vi "Send home.vi"(8 "error in (no error)":errorcluster, 11 "FCR Mod ID":i32) -> (0 "error out":errorcluster, 3 "Home?":bool)   [LabVIEW 2020]
uses:
  Newport_FCR100/Libraries/FCR100/Support/Device state -- enum.ctl
  Newport_FCR100/Libraries/FCR100/FCR100.lvlib
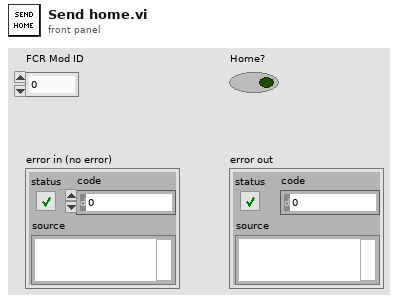
[diagram p1: front panel]
types:
  T1 = typedef "FCR100.lvlib/Device state -- enum.ctl" = enum16{"Not referenced", "Configuration", "Disable", "Ready", "Homing", "Motion"}
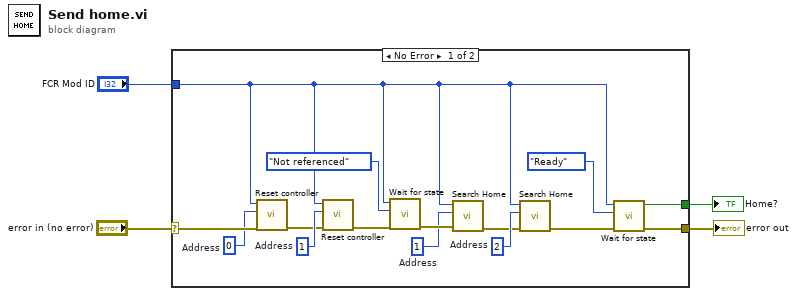
[diagram p0: block diagram]
diagram:
  n1 = case shown="No Error" "error in (no error)" {
    selector: "error in (no error)" -> [w17 w20]
    tunnel: "FCR Mod ID" -> [w19 _]
    tunnel: [w11 _] -> w2
    tunnel: [w9 w20] -> w1
    frame No Error {
      w15 = u8 1  # Address
      w16 = u8 0  # Address
      w7 = u8 2  # Address
      w5 = u8 1  # Address
      n2 = call "Reset controller.vi"("error in"=w17, "Address"=w16, "Module ID"=w19) -> ("error out"=w12:errorcluster)  [unwired: 8 in]
      n3 = call "Reset controller.vi"("error in"=w12, "Address"=w15, "Module ID"=w19) -> ("error out"=w13:errorcluster)  [unwired: 8 in]
      n4 = call "Wait for state.vi"("error in (no error)"=w13, "State"=Device_state_--_enum."Not referenced", "FCR Mod ID"=w19) -> ("error out"=w18:errorcluster)  [unwired: 7 in, 1 out]
      n5 = call "Search Home.vi"("error in"=w18, "Address"=w5, "Module ID"=w19) -> ("error out"=w6:errorcluster)  [unwired: 8 in]
      n6 = call "Search Home.vi"("error in"=w6, "Address"=w7, "Module ID"=w19) -> ("error out"=w8:errorcluster)  [unwired: 8 in]
      n7 = call "Wait for state.vi"("error in (no error)"=w8, "State"=Device_state_--_enum."Ready", "FCR Mod ID"=w19) -> ("error out"=w9:errorcluster, "Home?"=w11:bool)  [unwired: 7 in]
    }
    frame Error {
    }
  }
  "Home?" <- w2
  "error out" <- w1
